vi "Drop Parameters.vi"(6 "Main UI Message Queue":refnum<queue>, 7 "Mouse Position":cluster{"X":i32, "Y":i32}, 8 "error in (no error)":errorcluster, 9 "Parent Window Title":string, 10 "Module Type":T1=enum."Feed", 11 "State in":T2 {"Main Config"."PR Module Configs"."Settings"."PID 2 Parameters"."output range"."output low" format="%.2f"; "Main Config"."PR Module Configs"."Settings"."PID 2 Parameters"."output range"."output high" min=0.0 max=100.0 format="%.2f"; "Main Config"."PR Module Configs"."Settings"."PID 2 Parameters"."PID gains"."derivative time (Td, min)" format="%.3f"; "Main Config"."PR Module Configs"."Settings"."PID 2 Parameters"."PID gains"."integral time (Ti, min)" format="%.3f"; "Main Config"."PR Module Configs"."Settings"."PID 2 Parameters"."PID gains"."proportional gain (Kc)" format="%.3f"; "Main Config"."Steps"."Control" items=["Pump %", "Setpoint"]; "Main Config"."TCU Module Configs"."Settings"."Julabo FP-50 Settings"."Pump Power" min=0 max=8 step=1; "Main Config"."TCU Module Configs"."Settings"."Lauda Settings"."Pump Power" min=0 max=8 step=1; "Main Config"."Pump Module Configs"."Settings"."ASIA Pump C"."channel" min=0 max=1 step=1; "Main Config"."Pump Module Configs"."Settings"."Masterflex"."Pump Number" min=1.0 max=20.0 step=1.0; "Main Config"."Pump Module Configs"."Settings"."Ismatech"."Pump Number" min=1.0 max=20.0 step=1.0; "Main Config"."Feed Module Configs"."Settings"."output range"."output low" min=0.0 max=100.0 format="%.2f"; "Main Config"."Feed Module Configs"."Settings"."output range"."output high" format="%.2f"; "Main Config"."Feed Module Configs"."Settings"."PID 2 Parameters"."PID gains"."derivative time (Td, min)" format="%.3f"; "Main Config"."Feed Module Configs"."Settings"."PID 2 Parameters"."PID gains"."integral time (Ti, min)" format="%.3f"; "Main Config"."Feed Module Configs"."Settings"."PID 2 Parameters"."PID gains"."proportional gain (Kc)" format="%.3f"; "Main Config"."Feed Module Configs"."Settings"."ASIA Pump C"."channel" min=0 max=1 step=1; "Main Config"."Feed Module Configs"."Settings"."Ismatech"."Pump Number" min=1.0 max=20.0 step=1.0; "Main Config"."Feed Module Configs"."Settings"."Masterflex"."Pump Number" min=1.0 max=20.0 step=1.0}) -> (0 "error out":errorcluster, 2 "Drop Parameters":T63, 3 "State out":T2 {"Main Config"."PR Module Configs"."Settings"."PID 2 Parameters"."output range"."output low" format="%.2f"; "Main Config"."PR Module Configs"."Settings"."PID 2 Parameters"."output range"."output high" min=0.0 max=100.0 format="%.2f"; "Main Config"."PR Module Configs"."Settings"."PID 2 Parameters"."PID gains"."derivative time (Td, min)" format="%.3f"; "Main Config"."PR Module Configs"."Settings"."PID 2 Parameters"."PID gains"."integral time (Ti, min)" format="%.3f"; "Main Config"."PR Module Configs"."Settings"."PID 2 Parameters"."PID gains"."proportional gain (Kc)" format="%.3f"; "Main Config"."Steps"."Control" items=["Pump %", "Setpoint"]; "Main Config"."TCU Module Configs"."Settings"."Julabo FP-50 Settings"."Pump Power" min=0 max=8 step=1; "Main Config"."TCU Module Configs"."Settings"."Lauda Settings"."Pump Power" min=0 max=8 step=1; "Main Config"."Pump Module Configs"."Settings"."ASIA Pump C"."channel" min=0 max=1 step=1; "Main Config"."Pump Module Configs"."Settings"."Masterflex"."Pump Number" min=1.0 max=20.0 step=1.0; "Main Config"."Pump Module Configs"."Settings"."Ismatech"."Pump Number" min=1.0 max=20.0 step=1.0; "Main Config"."Feed Module Configs"."Settings"."output range"."output low" min=0.0 max=100.0 format="%.2f"; "Main Config"."Feed Module Configs"."Settings"."output range"."output high" format="%.2f"; "Main Config"."Feed Module Configs"."Settings"."PID 2 Parameters"."PID gains"."derivative time (Td, min)" format="%.3f"; "Main Config"."Feed Module Configs"."Settings"."PID 2 Parameters"."PID gains"."integral time (Ti, min)" format="%.3f"; "Main Config"."Feed Module Configs"."Settings"."PID 2 Parameters"."PID gains"."proportional gain (Kc)" format="%.3f"; "Main Config"."Feed Module Configs"."Settings"."ASIA Pump C"."channel" min=0 max=1 step=1; "Main Config"."Feed Module Configs"."Settings"."Ismatech"."Pump Number" min=1.0 max=20.0 step=1.0; "Main Config"."Feed Module Configs"."Settings"."Masterflex"."Pump Number" min=1.0 max=20.0 step=1.0})   [LabVIEW 2018, in "Drag and Drop.lvlib"]
uses:
  Drag and Drop.lvlib
  Drop Parameters Cluster.ctl
  support/Message Queue/Message Cluster.ctl
  <vilib>/Utility/miscctls.llb/LVPoint32TypeDef.ctl
  State Cluster.ctl
  Thumbnail Cluster.ctl
  Object Cluster.ctl
  <vilib>/Utility/miscctls.llb/LVRectTypeDef.ctl
  Object Type Enum.ctl
  <vilib>/Utility/miscctls.llb/LVPositionTypeDef.ctl
  Config Module/Controls/Main Config Cluster.ctl
  OPC/OPC Module Config.ctl
  Scale Module Folder/Measure Instrument/State Enum.ctl
  OPC/OPC Settings.ctl
  OPC/Variable Data Cluster.ctl
  <vilib>/OPCUA/controls/NodeId.ctl
  <vilib>/OPCUA/controls/OPC UA StatusCode.ctl
  <vilib>/OPCUA/controls/Subscription ID.ctl
  <vilib>/OPCUA/controls/OPC UA Client Refnum.ctl
  <vilib>/OPCUA/controls/Subscription Data Change.ctl
  <vilib>/OPCUA/controls/Data Type.ctl
  Feed Module/Controls/Feed Module Config Cluster.ctl
  Feed Module/Controls/Feed Module Settings Cluster.ctl
  Ismatec ISM 831C/Controls/Ismatech Settings Cluster.ctl
  Masterflex 7550-30/Controls/Settings Cluster.ctl
  Mettler Toledo/Controls/Settings Cluster.ctl
  Bronkhorst M13 Flow Meter/Settings Cluster.ctl
  Measure Instrument/PID 2 Parameters Cluster.ctl
  Measure Instrument/PID Input Enum.ctl
  Measure Instrument/PID 2 Output Enum.ctl
  Tacmina QI/Tacmina QI DAQ Setting.ctl
  KNF Pump/Settings Cluster plus SIMDOS.ctl
  ASIA Pump/Pump Settings.ctl
  VICI M50 Party Mode/Settings Cluster.ctl
  FLOM Pump/Settings Cluster.ctl
  SSI PR Class/SSI PR Settings Cluster.ctl
  TT Module/Controls/TT Module Config Cluster.ctl
  Acquisition/Hardware Configuration.ctl
  Acquisition/Task Cluster.ctl
  PT Module/Controls/PT Module Config Cluster.ctl
  Scale Module Folder/Feed Module/Controls/Scale Module Config Cluster.ctl
  Scale Module Folder/Feed Module/Controls/Scale Module Settings Cluster.ctl
  Pump Module Folder/Pump Module Config Cluster.ctl
  Pump Module Folder/Pump Module Settings Cluster.ctl
  LabJack Module/Controls/U3 Module Config Cluster.ctl
  Decoration Module/Decoration Module Config Cluster.ctl
  Flow Module Folder/Feed Module/Controls/Flow Module Config Cluster.ctl
  Flow Module Folder/Feed Module/Controls/Flow Module Settings Cluster.ctl
  TCU Module/TCU Module Folder/TCU Module Config Cluster.ctl
  TCU Module/TCU Module Folder/TCU Module Settings Cluster.ctl
  TCU Module/TCU Module Folder/Measure Instrument/Output Devices.ctl
  Huber TCU/Huber Settings.ctl
  Lauda Integral XT-150 TCU/Lauda Settings.ctl
  Julabo Type 1 TCU/Julabo Type 1 TCU Folder/Julabo FP-50 Settings.ctl
  Huber Unistat 410 TCU/Huber Unistat 410 Settings.ctl
  D-O Module Folder/Not Sure Where this is Used.ctl
  Sequencing/Squence Control.ctl
  D-O Module Folder/D-O Module Config Cluster.ctl
  D-O Module Folder/Valve Clusters.ctl
  D-O Module Folder/D-O Module Settings Cluster.ctl
  D-O Module Folder/D-O Device Settings Cluster.ctl
  VICI Electronic Actuator/VICI Electronic Actuator Settings.ctl
  Pressure Regulator Control Module/Pressure Regulator/Controls/4-20mA Module Config Cluster.ctl
  Pressure Regulator Control Module/Pressure Regulator/Controls/4-20mA Module Settings Cluster.ctl
  Pressure Transmitter/Pressure Transmitter Device Settings.ctl
  Pressure Reg Module/Pressure Regulator Device Settings.ctl
  Module Type Enum.ctl
  Module Instance Number Operation Enum.ctl
  Flow Module Folder/Flow Module (Main).vi
  D-O Module Folder/D-O Module (Main).vi
  TCU Module/TCU Module Folder/TCU Module (Main).vi
  LabJack Module/U3 (Main).vit
  Feed Module/Feed Module.lvlib
  TT Module/TT Module.lvlib
  support/Message Queue/Message Queue.lvlib
  Bronkhorst M13 Flow Meter/Bronkhorst M13 Flow Meter.lvlib
  Mettler Toledo/Mettler Toledo.lvlib
  Masterflex 7550-30/Masterflex 7550-30.lvlib
  Ismatec ISM 831C/Ismatec ISM 831C.lvlib
  PT Module/PT Module.lvlib
  Shared Variables/Dynamic Shared Variables.lvlib
  Scale Module Folder/Scale Module.lvlib
  Pump Module Folder/Pump Module.lvlib
  LabJack Module/U3 Module.lvlib
  Flow Module Folder/Flow Module.lvlib
  Tacmina QI/Tacmina QI.lvlib
  KNF Pump/KNF SIMDOS.lvlib
  TCU Module/TCU Module Folder/TCU Module.lvlib
  Huber TCU/Huber Ministat 230 TCU.lvlib
  Lauda Integral XT-150 TCU/Lauda TCU.lvlib
  Julabo Type 1 TCU/Julabo Type 1 TCU Folder/Julabo Type FP-50 TCU.lvlib
  ASIA Pump.lvlib
  VICI M50 Party Mode/VICI M6 M50 Party Mode.lvlib
  D-O Module Folder/D-O Module.lvlib
  Pressure Regulator Control Module/Pressure Regulator/4-20mA Module.lvlib
  Pressure Transmitter/Pressure Transmitter Library.lvlib
  Pressure Reg Module/Pressure Regulator Library.lvlib
  FLOM Pump/FLOM Pump.lvlib
  SSI PR Class/SSI PR Pump.lvlib
  Huber Unistat 410 TCU/Huber Unistat 410 TCU.lvlib
  OPC/OPC UA.lvlib
  Scale Module Folder/Measure Instrument/Scale Module Engine.lvlib
  D-O Module Folder/DIO Valve/VICI Electronic Actuator.lvlib
  D-O Module Folder/D-O Module (Main) 2nd.vi
  Config Module/Config Module.lvlib
  DAQ/DAQ.lvlib
  Sequencing/Sequencing Library.lvlib
panel:
  # "Instrument Settings"
  # "Instrument Settings"
  # "Output Instruments"
  # "Flow Meter Settings"
  # "Output Instruments"
  # "Scale Settings"
  # "Output Instruments"
  # "Input Instruments"
  # "Instrument Settings"
  # "Instrument Settings"
  # "Output Instruments"
  # "Flow Meter Settings"
  # "Output Instruments"
  # "Scale Settings"
  # "Output Instruments"
  # "Input Instruments"
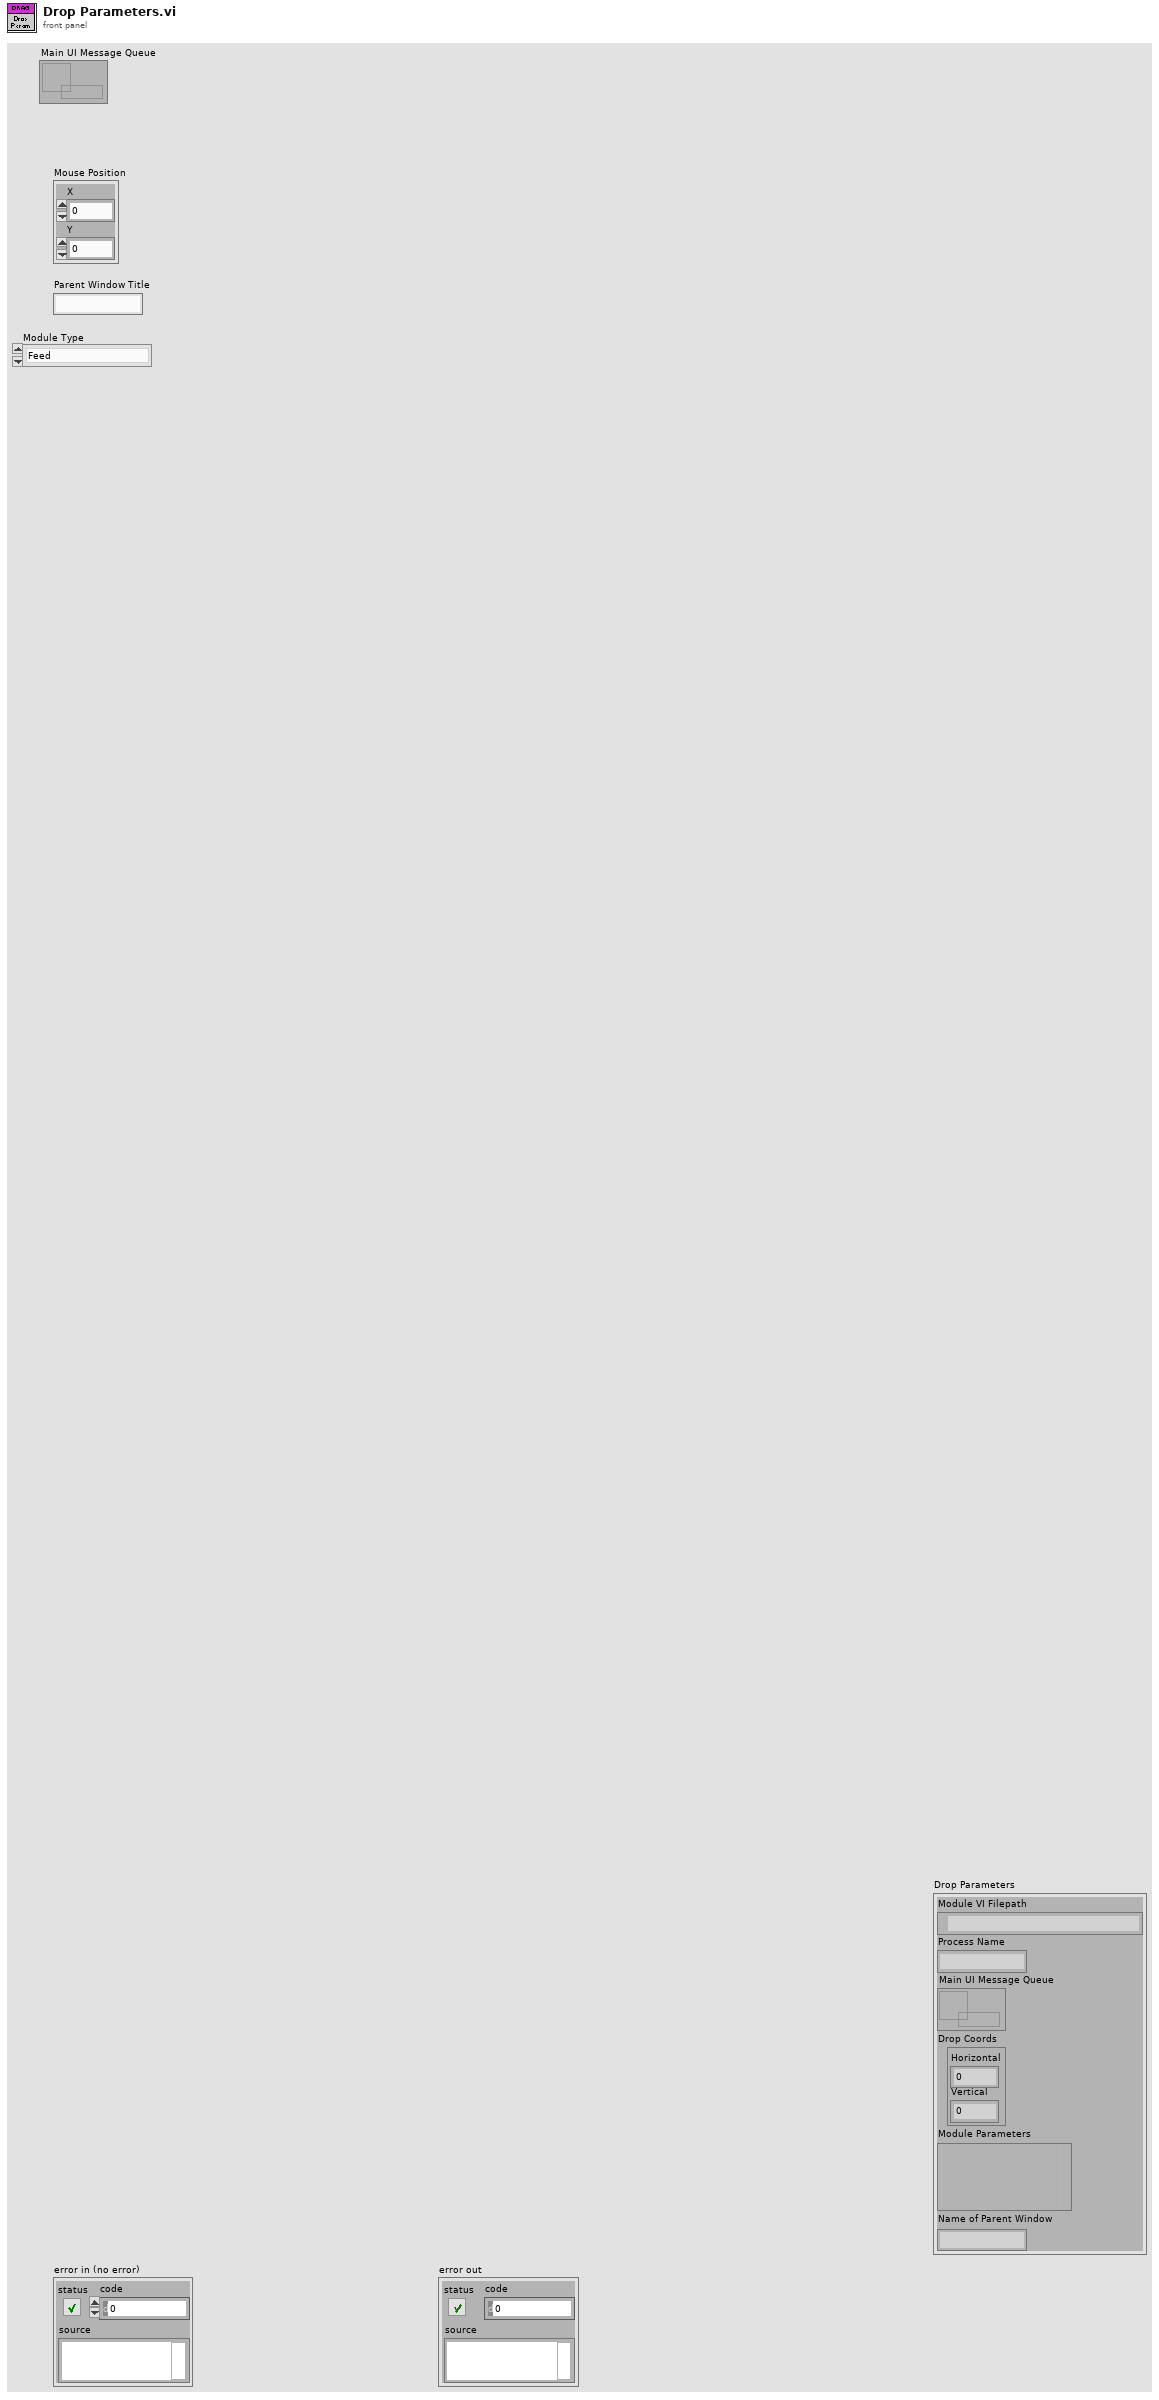
[diagram p1: front panel]
types:
  T1 = typedef "Drag and Drop.lvlib/Module Type Enum.ctl" = enum16{"<unknown module>", "Feed", "TT", "PT", "Scale", "Flow", "Pump", "U3", "TCU", "DO", "PR", "OPC"}
  T2 = typedef "Drag and Drop.lvlib/State Cluster.ctl" = cluster{"VI refs":refnum<vi>[], "Queues":refnum<queue>[], "[Thumbnails]":T3[], "Drag Object Idx":i32, "[Objects]":T4[], "Active Object":i32, "Drop Offset":T7, "Process Name":string, "Main Config":T8, "Campaign Filepath":path, "Config Changed?":bool}
  T3 = typedef "Thumbnail Cluster.ctl" = cluster{"Path":path, "Rectangle":cluster{"left":i16, "top":i16, "right":i16, "bottom":i16}}
  T4 = typedef "Object Cluster.ctl" = cluster{"BMP Path":path, "Anchor Position":cluster{"X":i32, "Y":i32}, "Hot Spot":T5, "Type":T6, "Parameters":variant}
  T5 = typedef "LVRectTypeDef.ctl" = cluster{"Left":i16, "Top":i16, "Right":i16, "Bottom":i16}
  T6 = typedef "Object Type Enum.ctl" = enum16{"Icon", "Line", "Text", "Feed Module"}
  T7 = typedef "LVPositionTypeDef.ctl" = cluster{"Left":i32, "Top":i32}
  T8 = typedef "Config Module.lvlib/Main Config Cluster.ctl" = cluster{"OPC Module Configs":T9[], "Feed Module Configs":T18[], "Log File Path":path, "TT Module Configs":T33[], "DAQ Config":T34, "PT Module Configs":T36[], "Scale Module Configs":T37[], "Pump Module Configs":T39[], "U3 Module Configs":T41[], "Decoration Module Configs":T42[], "Flow Module Configs":T43[], "TCU Module Configs":T45[], "Steps":T52, "Abort":bool, "DO Module Configs":T54[], "PR Module Configs":T59[], "Cycle Period":dbl}
  T9 = typedef "OPC UA.lvlib/OPC Module Config.ctl" = cluster{"State":T10, "GUID":string, "Drop Coords":T11, "Configuration":T12, "First Iteration":bool, "Data":cluster{"Object Name":string, "Variable Array":T13[]}[], "Process Name":string, "Load Count":i32, "Log Started":bool, "subscription ID out":T16, "OPC UA client refnum out":T17, "Event Registration Refnum":refnum<event-registration>, "Start Time":timestamp, "Current Time":timestamp}
  T10 = typedef "Scale Module.lvlib/Scale Module Engine.lvlib/State Enum.ctl" = enum16{"Measuring", "Idle"}
  T11 = typedef "LVPoint32TypeDef.ctl" = cluster{"Horizontal":i32, "Vertical":i32}
  T12 = typedef "OPC UA.lvlib/OPC Settings.ctl" = cluster{"Cycle Period":dbl, "server endpoint URL":string, "security policy":cluster{"message mode":enum16{"None", "Sign", "Sign and Encrypt"}, "security":enum16{"Basic256", "Basic128Rsa15"}}, "Trust Any Server":bool}
  T13 = typedef "OPC UA.lvlib/Variable Data Cluster.ctl" = cluster{"node ID":T14, "browse name":string, "status":T15, "timestamp":timestamp, "value ":variant}
  T14 = typedef "NodeId.ctl" = string
  T15 = typedef "OPC UA StatusCode.ctl" = u32
  T16 = typedef "Subscription ID.ctl" = u32
  T17 = typedef "OPC UA Client Refnum.ctl" = refnum<k21>
  T18 = typedef "Feed Module.lvlib/Feed Module Config Cluster.ctl" = cluster{"GUID":string, "Drop Coords":T11, "Process Name":string, "Queue Name":string, "Settings":T19, "Settings Load Count":i32, "OP Load Count":i32}
  T19 = typedef "Feed Module.lvlib/Feed Module Settings Cluster.ctl" = cluster{"Cycle Period":dbl, "Ismatech":T20, "Masterflex":T21, "Mettler":T22, "Bronkhorst M13 Flow Meter":T23, "PID 2 Parameters":T24, "Manual Entry":dbl, "Auto?":bool, "output range":cluster{"output high":dbl, "output low":dbl}, "Bronkhorst M14":T22, "Tacmina Settings":T27, "KNF SIMDOS Settings":T28, "ASIA Pump C":T29, "VICI Settings":T30, "FLOM Settings":T31, "SSI PR Settings":T32}
  T20 = typedef "Ismatec ISM 831C.lvlib/Ismatech Settings Cluster.ctl" = cluster{"VISA resource name":refnum<visa-resource-name>, "Simulated?":bool, "Pump Number":dbl, "Reverse?":bool}
  T21 = typedef "Masterflex 7550-30.lvlib/Settings Cluster.ctl" = cluster{"VISA resource name":refnum<visa-resource-name>, "Simulated?":bool, "Pump Number":dbl, "Reverse?":bool}
  T22 = typedef "Mettler Toledo.lvlib/Settings Cluster.ctl" = cluster{"VISA resource name":refnum<visa-resource-name>, "Simulated?":bool}
  T23 = typedef "Bronkhorst M13 Flow Meter.lvlib/Settings Cluster.ctl" = cluster{"VISA resource name":refnum<visa-resource-name>, "Simulated?":bool}
  T24 = typedef "PID 2 Parameters Cluster.ctl" = cluster{"Input Device":T25, "Output Device":T26, "Setpoint":dbl, "PID gains":cluster{"proportional gain (Kc)":dbl, "integral time (Ti, min)":dbl, "derivative time (Td, min)":dbl}}
  T25 = typedef "PID Input Enum.ctl" = enum16{"Default", "Bronkhorst M13", "Bronkhorst M14", "Scale Rate of Change"}
  T26 = typedef "PID 2 Output Enum.ctl" = enum16{"Default", "Ismatec ISM 831C", "Masterflex 7550-30", "VICI", "Tacmina QI", "KNF SIMDOS", "ASIA Type C", "FLOM UI-22-11", "SSI PR"}
  T27 = typedef "Tacmina QI.lvlib/Tacmina QI DAQ Setting.ctl" = cluster{"Analog DAQ Task":refnum<k21>, "Digital DAQ Task":refnum<k21>}
  T28 = typedef "KNF SIMDOS.lvlib/Settings Cluster plus SIMDOS.ctl" = cluster{"VISA resource name":refnum<visa-resource-name>, "Simulated?":bool}
  T29 = typedef "ASIA Pump.lvlib/Pump Settings.ctl" = cluster{"ASIA Pump #":i32, "channel":i32, "Simulated":bool}
  T30 = typedef "VICI M6 M50 Party Mode.lvlib/Settings Cluster.ctl" = cluster{"VISA resource name":refnum<visa-resource-name>, "Simulated?":bool, "Pump Letter":string, "Reverse?":bool}
  T31 = typedef "FLOM Pump.lvlib/Settings Cluster.ctl" = cluster{"VISA resource name":refnum<visa-resource-name>, "Simulated?":bool, "Pump Number":dbl}
  T32 = typedef "SSI PR Pump.lvlib/SSI PR Settings Cluster.ctl" = cluster{"VISA resource name":refnum<visa-resource-name>, "Simulated?":bool}
  T33 = typedef "TT Module.lvlib/TT Module Config Cluster.ctl" = cluster{"GUID":string, "Drop Coords":T11, "Input Channel Tag Name ":string, "Process Name":string, "Queue Name":string, "Input Channel Numeric Alarm Settings":cluster{"enable? (F)":bool, "name":string, "alarm type":enum16{"HI_HI", "HI", "LO", "LO_LO"}, "level/change":dbl, "deadband/time":dbl, "priority":u32, "ack type":enum16{"Auto", "User", "None", "Each Occurrence"}, "area":string, "description":string, "log? (T)":bool}[]}
  T34 = typedef "DAQ.lvlib/Hardware Configuration.ctl" = cluster{"Tasks":T35[]}
  T35 = typedef "Task Cluster.ctl" = cluster{"DAQmx Task":refnum<k21>, "Read-Write Radio":enum32{"Read", "Write"}}
  T36 = typedef "PT Module.lvlib/PT Module Config Cluster.ctl" = cluster{"GUID":string, "Drop Coords":T11, "Input Channel Tag Name ":string, "Process Name":string, "Queue Name":string, "Input Channel Numeric Alarm Settings":cluster{"enable? (F)":bool, "name":string, "alarm type":enum16{"HI_HI", "HI", "LO", "LO_LO"}, "level/change":dbl, "deadband/time":dbl, "priority":u32, "ack type":enum16{"Auto", "User", "None", "Each Occurrence"}, "area":string, "description":string, "log? (T)":bool}[]}
  T37 = typedef "Scale Module.lvlib/Scale Module Config Cluster.ctl" = cluster{"GUID":string, "Drop Coords":T11, "Process Name":string, "Queue Name":string, "Settings":T38, "Load Count":i32}
  T38 = typedef "Scale Module.lvlib/Scale Module Settings Cluster.ctl" = cluster{"Cycle Period":dbl, "Mettler":T22, "Scale Type":string}
  T39 = typedef "Pump Module.lvlib/Pump Module Config Cluster.ctl" = cluster{"GUID":string, "Drop Coords":T11, "Process Name":string, "Queue Name":string, "Settings":T40, "Load Count":i32}
  T40 = typedef "Pump Module.lvlib/Pump Module Settings Cluster.ctl" = cluster{"Cycle Period":dbl, "Ismatech":T20, "Masterflex":T21, "Manual Entry":dbl, "VICI Settings":T30, "Output Device":T26, "Tacmina Settings":T27, "KNF SIMDOS Settings":T28, "ASIA Pump C":T29, "FLOM Settings":T31, "Pump Calibration File":path, "Calibration":dbl, "Pump Cal Enum":u16, "SSI PR Settings":T32}
  T41 = typedef "U3 Module.lvlib/U3 Module Config Cluster.ctl" = cluster{"GUID":string, "Drop Coords":T11, "AI Channel Number":enum16{"Default", "AI0", "AI1", "AI2", "AI3", "AI4", "AI5", "AI6", "AI7"}, "Process Name":string, "Queue Name":string, "Input Channel Numeric Alarm Settings":cluster{"enable? (F)":bool, "name":string, "alarm type":enum16{"HI_HI", "HI", "LO", "LO_LO"}, "level/change":dbl, "deadband/time":dbl, "priority":u32, "ack type":enum16{"Auto", "User", "None", "Each Occurrence"}, "area":string, "description":string, "log? (T)":bool}[]}
  T42 = typedef "Decoration Module Config Cluster.ctl" = cluster{"GUID":string, "Drop Coords":T11, "Decoration Filepath":path}
  T43 = typedef "Flow Module.lvlib/Flow Module Config Cluster.ctl" = cluster{"GUID":string, "Drop Coords":T11, "Process Name":string, "Queue Name":string, "Settings":T44, "Load Count":i32}
  T44 = typedef "Flow Module.lvlib/Flow Module Settings Cluster.ctl" = cluster{"Cycle Period":dbl, "Bronkhorst M13":T22, "Flow Meter Type":string, "Bronkhorst M14":T22}
  T45 = typedef "TCU Module.lvlib/TCU Module Config Cluster.ctl" = cluster{"GUID":string, "Drop Coords":T11, "Process Name":string, "Queue Name":string, "Settings":T46, "Load Count":i32, "Power Level Changed":bool}
  T46 = typedef "TCU Module.lvlib/TCU Module Settings Cluster.ctl" = cluster{"Cycle Period":dbl, "Setpoint Entry":dbl, "Output Device":T47, "Huber Ministat 230 Settings":T48, "Lauda Settings":T49, "Julabo FP-50 Settings":T50, "Internal Control?":bool, "Huber Unistat 410 Settings":T51}
  T47 = typedef "Output Devices.ctl" = enum16{"Default", "Huber Ministat 230", "Huber Unistat 410", "Lauda XT-150", "Julabo FP-50"}
  T48 = typedef "Huber Ministat 230 TCU.lvlib/Huber Settings.ctl" = cluster{"VISA resource name":refnum<visa-resource-name>, "Simulated?":bool}
  T49 = typedef "Lauda TCU.lvlib/Lauda Settings.ctl" = cluster{"VISA resource name":refnum<visa-resource-name>, "Simulated?":bool, "Pump Power":i32}
  T50 = typedef "Julabo Type FP-50 TCU.lvlib/Julabo FP-50 Settings.ctl" = cluster{"VISA resource name":refnum<visa-resource-name>, "Simulated?":bool, "Pump Power":i32}
  T51 = typedef "Huber Unistat 410 TCU.lvlib/Huber Unistat 410 Settings.ctl" = cluster{"VISA resource name":refnum<visa-resource-name>, "Simulated?":bool}
  T52 = typedef "Not Sure Where this is Used.ctl" = T53[]
  T53 = typedef "Sequencing Library.lvlib/Squence Control.ctl" = cluster{"Module":string, "Control":u16, "Value":dbl, "Wait (sec)":dbl}
  T54 = typedef "D-O Module.lvlib/D-O Module Config Cluster.ctl" = cluster{"GUID":string, "Drop Coords":T11, "Process Name":string, "Queue Name":string, "Settings":T55, "Load Count":i32}
  T55 = typedef "D-O Module.lvlib/Valve Clusters.ctl" = cluster{"Valve Settings":T56, "Valve Type":enum16{"Default", "Digital Output Valve", "VICI Electronic Actuator"}, "Time On (Sec)":dbl, "Time Off (Sec)":dbl, "Run?":bool}
  T56 = typedef "D-O Module.lvlib/D-O Module Settings Cluster.ctl" = cluster{"D-O Settings":T57, "VICI Electronic Actuator":T58}
  T57 = typedef "D-O Module.lvlib/D-O Device Settings Cluster.ctl" = cluster{"DAQmx Task Name":refnum<k21>, "Output Channel":u16, "Output Channel Names":string[]}
  T58 = typedef "VICI Electronic Actuator.lvlib/VICI Electronic Actuator Settings.ctl" = cluster{"VISA resource name":refnum<visa-resource-name>, "Mode":enum16{"Two Positions With Stops", "Two Positions Without Stops", "Mutiposition"}, "Simulated":bool}
  T59 = typedef "4-20mA Module.lvlib/4-20mA Module Config Cluster.ctl" = cluster{"GUID":string, "Drop Coords":T11, "Process Name":string, "Queue Name":string, "Settings":T60, "Settings Load Count":i32}
  T60 = typedef "4-20mA Module.lvlib/4-20mA Module Settings Cluster.ctl" = cluster{"Cycle Period":dbl, "PID 2 Parameters":cluster{"Input Device":enum16{"Default", "4-20mA"}, "Output Device":enum16{"Default", "Equilibar Pressure Reg", "Flow Regulator"}, "Setpoint":dbl, "PID gains":cluster{"proportional gain (Kc)":dbl, "integral time (Ti, min)":dbl, "derivative time (Td, min)":dbl}, "output range":cluster{"output low":dbl, "output high":dbl}}, "Manual Entry":dbl, "Auto?":bool, "4-20mA Input Settings":T61, "4-20mA Out Settings":T62, "Input Channel Tag Name ":string}
  T61 = typedef "Pressure Transmitter Library.lvlib/Pressure Transmitter Device Settings.ctl" = cluster{"Input Channel ":u16}
  T62 = typedef "Pressure Regulator Library.lvlib/Pressure Regulator Device Settings.ctl" = cluster{"Output DAQ Task":refnum<k21>}
  T63 = typedef "Drop Parameters Cluster.ctl" = cluster{"Module VI Filepath":path, "Process Name":string, "Main UI Message Queue":refnum<queue>, "Drop Coords":T11, "Module Parameters":variant, "Name of Parent Window":string}
  T64 = typedef "Module Instance Number Operation Enum.ctl" = enum16{"Init", "Next Instance Number"}
  T65 = cluster{"enable? (F)":bool, "name":string, "alarm type":enum16{"HI_HI", "HI", "LO", "LO_LO"}, "level/change":dbl, "deadband/time":dbl, "priority":u32, "ack type":enum16{"Auto", "User", "None", "Each Occurrence"}, "area":string, "description":string, "log? (T)":bool}[]
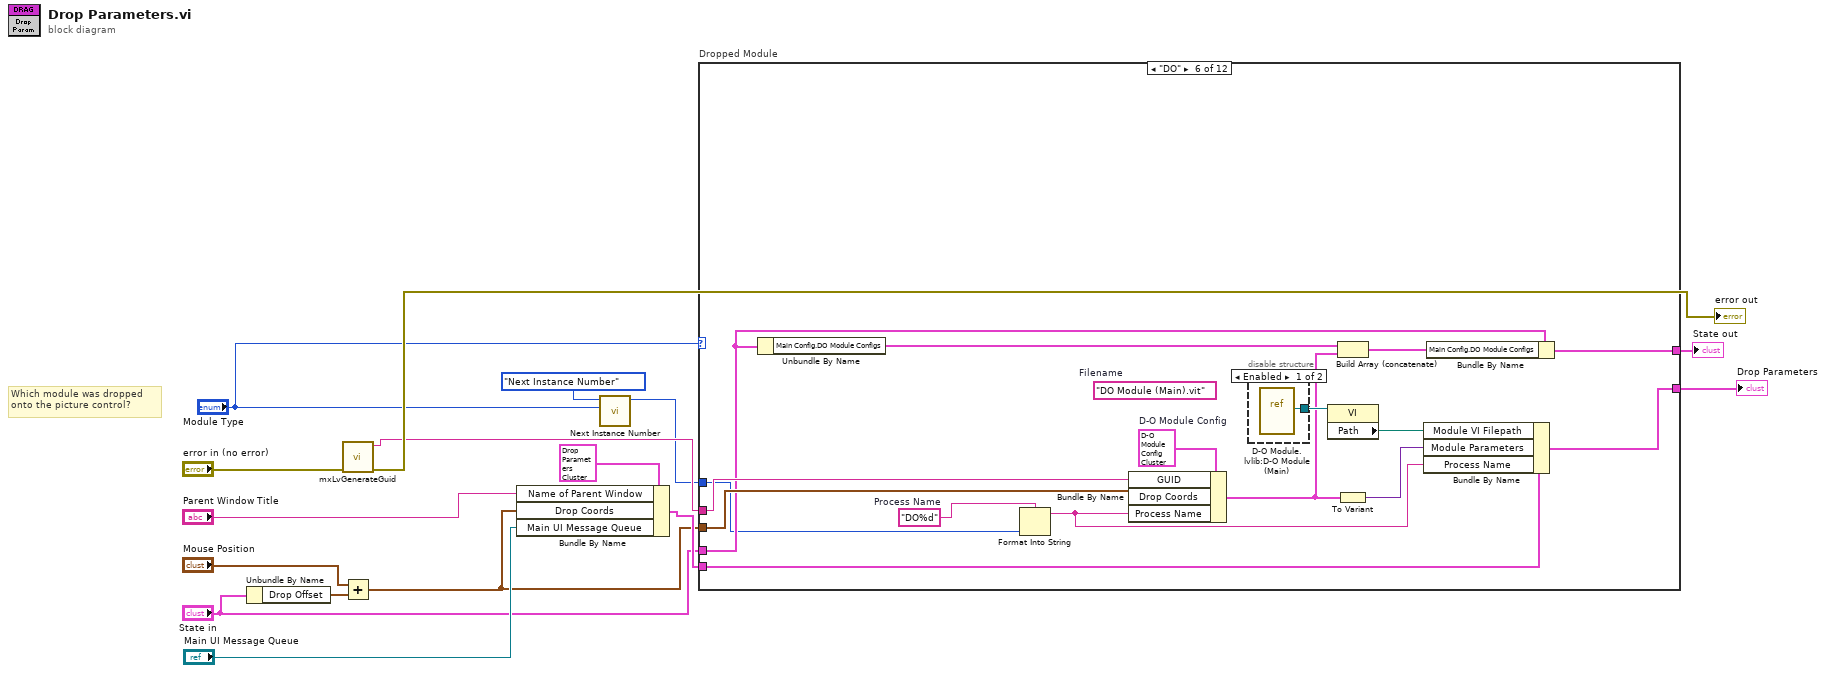
[diagram p0: block diagram]
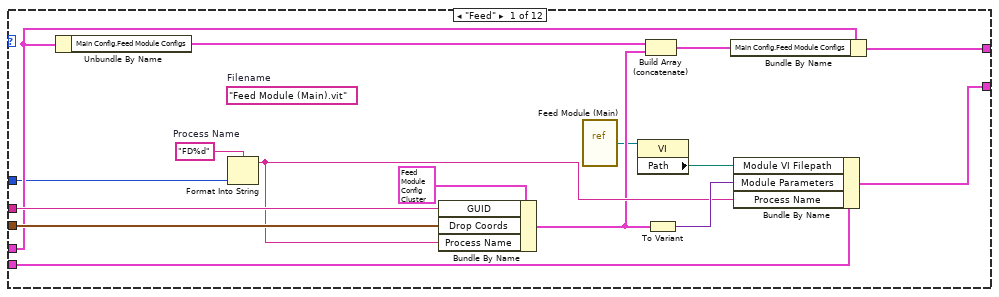
[diagram p2: hidden frame]
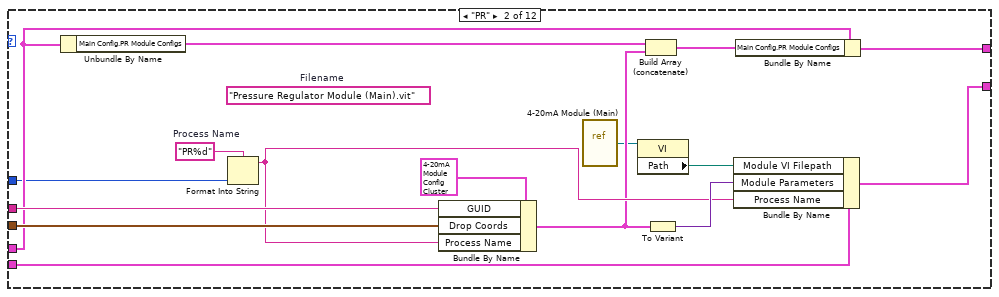
[diagram p3: hidden frame]
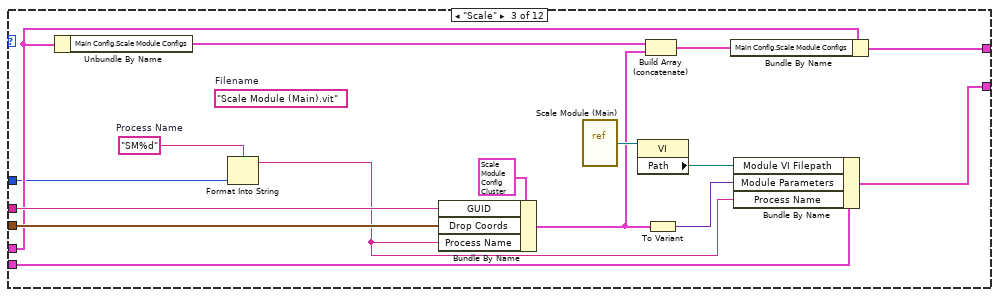
[diagram p4: hidden frame]
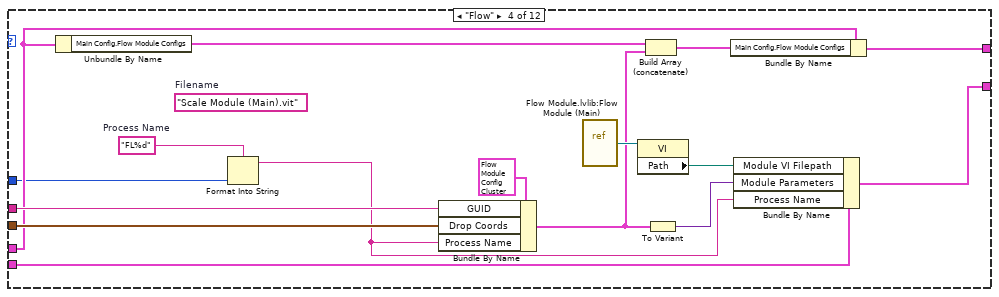
[diagram p5: hidden frame]
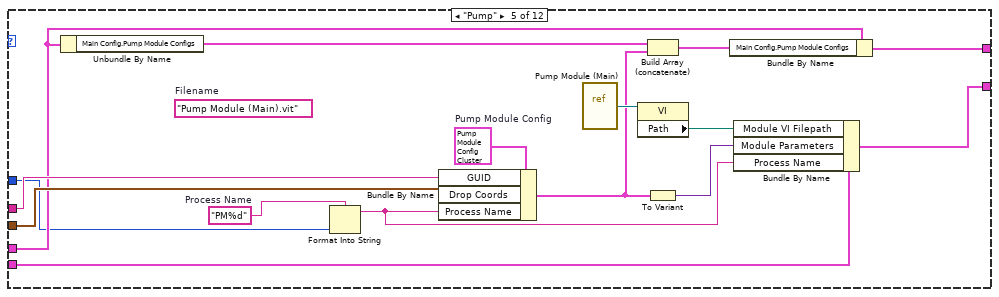
[diagram p6: hidden frame]
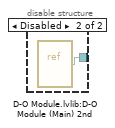
[diagram p7: hidden frame]
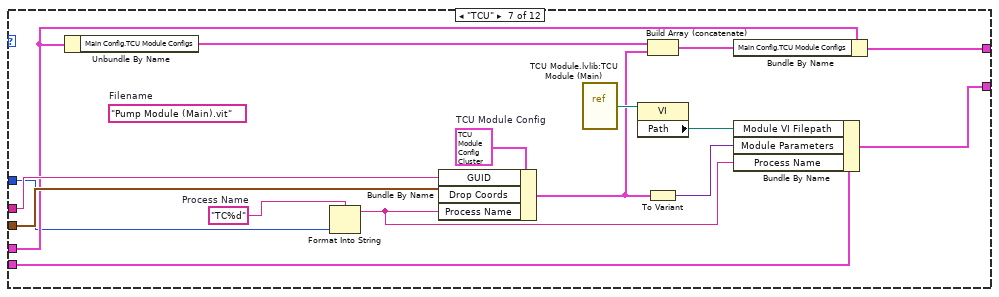
[diagram p8: hidden frame]
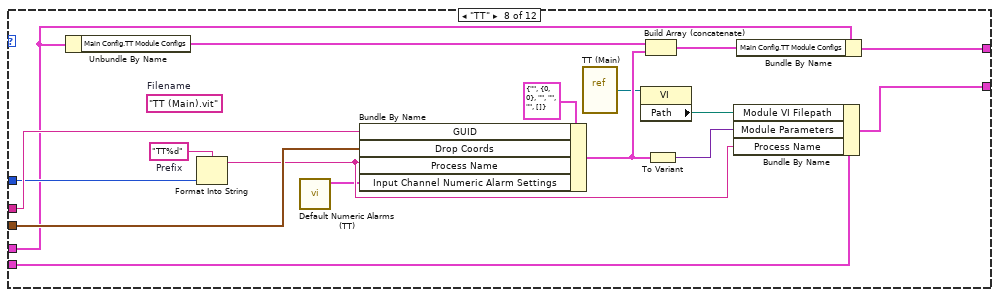
[diagram p9: hidden frame]
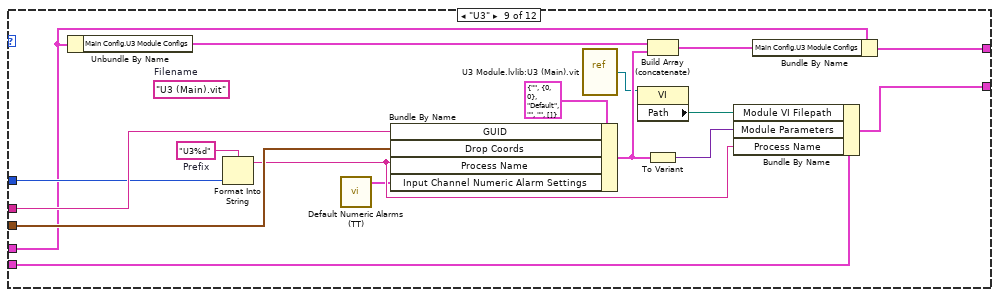
[diagram p10: hidden frame]
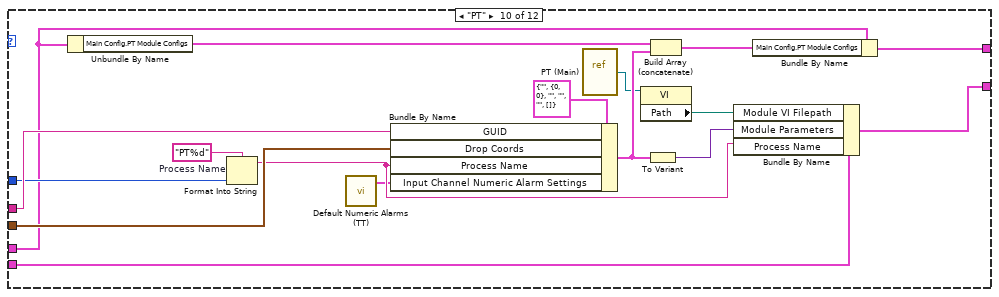
[diagram p11: hidden frame]
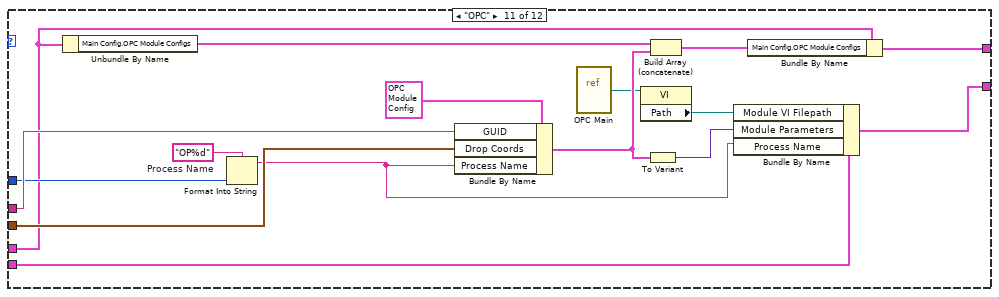
[diagram p12: hidden frame]
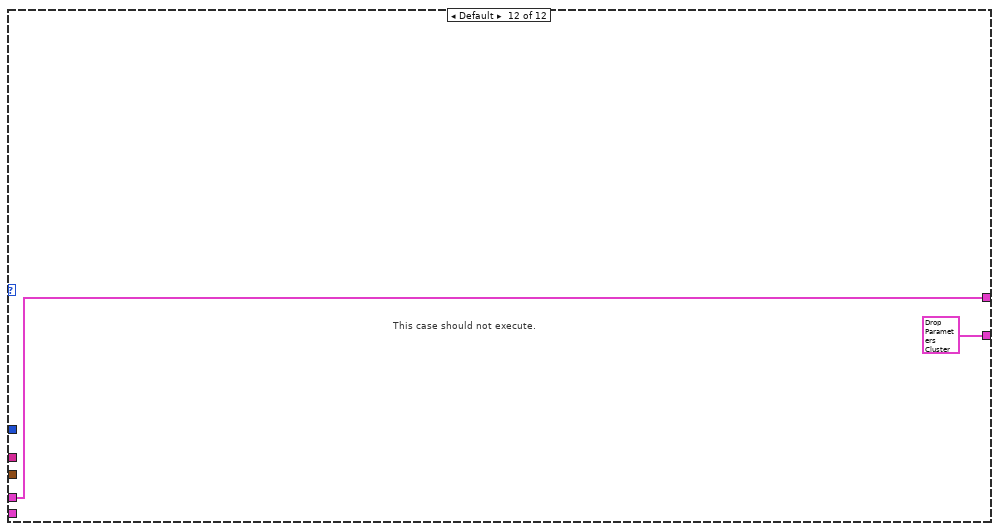
[diagram p13: hidden frame]
diagram:
  # "Which module was dropped\nonto the picture control?"
  n1 = Unbundle By Name("State in") -> ("Drop Offset"=w12:T7)
  n2 = call <resource>:"mxLvGenerateGuid.vi"("Error In"="error in (no error)") -> ("Error Out"=→"error out":errorcluster, "Value"=w13:string)  [unwired: 9 in]
  n3 = Add(x="Mouse Position", y=w12) -> (x+y=w6:T7)
  n4 = Bundle By Name(cluster=T63 {"Module VI Filepath"=path "", "Process Name"="", "Main UI Message Queue"=refnum, "Drop Coords"={"Horizontal"=0, "Vertical"=0}, "Module Parameters"=variant, "Name of Parent Window"=""} ("Drop Parameters"), "Name of Parent Window"="Parent Window Title", "Drop Coords"=w6, "Main UI Message Queue"="Main UI Message Queue") -> (w8:T63)
  n5 = call "Next Instance Number.vi"("Module Type"="Module Type", "Operation"=Module_Instance_Number_Operation_Enum."Next Instance Number") -> ("Instance Number"=w3:i32)  [unwired: 8 in, 1 out]
  n6 = case "Dropped Module" shown="\"DO\"" "Module Type" {
    tunnel: "State in" -> [w18 w34 w51 w67 w84 w100 w118 w132 w149 w166 w185 w199]
    tunnel: [w24 w40 w56 w72 w89 w105 w123 w136 w153 w170 w188 w199] -> w2
    tunnel: [w30 w46 w62 w78 w95 w111 w129 w146 w163 w180 w182 T63 {"Module VI Filepath"=path "", "Process Name"="", "Main UI Message Queue"=refnum, "Drop Coords"={"Horizontal"=0, "Vertical"=0}, "Module Parameters"=variant, "Name of Parent Window"=""} ("Drop Parameters")] -> w16
    tunnel: w13 -> [w29 w45 w61 w77 w94 w110 w128 w145 w162 w179 w196 _]
    tunnel: w8 -> [w28 w44 w60 w76 w93 w109 w127 w144 w161 w178 w195 _]
    tunnel: w6 -> [w26 w42 w58 w74 w91 w107 w125 w142 w159 w176 w193 _]
    tunnel: w3 -> [w17 w33 w50 w66 w83 w99 w117 w133 w150 w167 w186 _]
    frame "Feed" {
      w31 = "FD%d"  # Process Name
      (unwired) "Feed Module (Main).vit"  # Filename
      n7 = Unbundle By Name(w18) -> ("Main Config.Feed Module Configs"=w23:T18[])
      n8 = Format Into String(format string=w31, w17) -> (resulting string=w25:string)  [unwired: 2 in, 1 out]
      n9 = Bundle By Name(cluster=T18 {"GUID"="", "Drop Coords"={"Horizontal"=0, "Vertical"=0}, "Process Name"="", "Queue Name"="", "Settings"={"Cycle Period"=500.0, "Ismatech"={"VISA resource name"="", "Simulated?"=TRUE, "Pump Number"=1.0, "Reverse?"=FALSE}, "Masterflex"={"VISA resource name"="", "Simulated?"=TRUE, "Pump Number"=1.0, "Reverse?"=FALSE}, "Mettler"={"VISA resource name"="", "Simulated?"=FALSE}, "Bronkhorst M13 Flow Meter"={"VISA resource name"="", "Simulated?"=TRUE}, "PID 2 Parameters"={"Input Device"=enum."Default", "Output Device"=enum."Default", "Setpoint"=0.0, "PID gains"={"proportional gain (Kc)"=1.0, "integral time (Ti, min)"=0.01, "derivative time (Td, min)"=0.0}}, "Manual Entry"=0.0, "Auto?"=TRUE, "output range"={"output high"=100.0, "output low"=0.0}, "Bronkhorst M14"={"VISA resource name"="", "Simulated?"=FALSE}, "Tacmina Settings"={"Analog DAQ Task"="", "Digital DAQ Task"=""}, "KNF SIMDOS Settings"={"VISA resource name"="", "Simulated?"=TRUE}, "ASIA Pump C"={"ASIA Pump #"=0, "channel"=0, "Simulated"=FALSE}, "VICI Settings"={"VISA resource name"="", "Simulated?"=TRUE, "Pump Letter"="", "Reverse?"=FALSE}, "FLOM Settings"={"VISA resource name"="", "Simulated?"=TRUE, "Pump Number"=0.0}, "SSI PR Settings"={"VISA resource name"="", "Simulated?"=FALSE}}, "Settings Load Count"=0, "OP Load Count"=0} ("Feed Module Config"), "GUID"=w29, "Drop Coords"=w26, "Process Name"=w25) -> (w21:T18)
      n10 = vi-ref "Feed Module (Main).vi"() -> (w20:refnum<vi>)
      n11 = property class="VI"(reference=w20) -> ("Path"=w19:path)  [unwired: 1 in, 2 out]
      n12 = Build Array (concatenate)(w23, w21) -> (w22:T18[])
      n13 = To Variant(anything=w21) -> (Variant=w27:variant)
      n14 = Bundle By Name(cluster=w18, "Main Config.Feed Module Configs"=w22) -> (w24:T2)
      n15 = Bundle By Name(cluster=w28, "Module VI Filepath"=w19, "Module Parameters"=w27, "Process Name"=w25) -> (w30:T63)
    }
    frame "PR" {
      w47 = "PR%d"  # Process Name
      (unwired) "Pressure Regulator Module (Main).vit"  # Filename
      n16 = Unbundle By Name(w34) -> ("Main Config.PR Module Configs"=w39:T59[])
      n17 = Format Into String(format string=w47, w33) -> (resulting string=w41:string)  [unwired: 2 in, 1 out]
      n18 = Bundle By Name(cluster=T59 {"GUID"="", "Drop Coords"={"Horizontal"=0, "Vertical"=0}, "Process Name"="", "Queue Name"="", "Settings"={"Cycle Period"=500.0, "PID 2 Parameters"={"Input Device"=enum."Default", "Output Device"=enum."Default", "Setpoint"=0.0, "PID gains"={"proportional gain (Kc)"=1.0, "integral time (Ti, min)"=0.01, "derivative time (Td, min)"=0.0}, "output range"={"output low"=0.0, "output high"=100.0}}, "Manual Entry"=0.0, "Auto?"=TRUE, "4-20mA Input Settings"={"Input Channel "=0}, "4-20mA Out Settings"={"Output DAQ Task"=""}, "Input Channel Tag Name "=""}, "Settings Load Count"=0} ("PRM Config"), "GUID"=w45, "Drop Coords"=w42, "Process Name"=w41) -> (w37:T59)
      n19 = vi-ref "4-20mA Module (Main).vi"() -> (w36:refnum<vi>)
      n20 = property class="VI"(reference=w36) -> ("Path"=w35:path)  [unwired: 1 in, 2 out]
      n21 = Build Array (concatenate)(w39, w37) -> (w38:T59[])
      n22 = To Variant(anything=w37) -> (Variant=w43:variant)
      n23 = Bundle By Name(cluster=w44, "Module VI Filepath"=w35, "Module Parameters"=w43, "Process Name"=w41) -> (w46:T63)
      n24 = Bundle By Name(cluster=w34, "Main Config.PR Module Configs"=w38) -> (w40:T2)
    }
    frame "Scale" {
      w63 = "SM%d"  # Process Name
      (unwired) "Scale Module (Main).vit"  # Filename
      n25 = Unbundle By Name(w51) -> ("Main Config.Scale Module Configs"=w55:T37[])
      n26 = Format Into String(format string=w63, w50) -> (resulting string=w57:string)  [unwired: 2 in, 1 out]
      n27 = Bundle By Name(cluster=T37 {"GUID"="", "Drop Coords"={"Horizontal"=0, "Vertical"=0}, "Process Name"="", "Queue Name"="", "Settings"={"Cycle Period"=500.0, "Mettler"={"VISA resource name"="", "Simulated?"=TRUE}, "Scale Type"=""}, "Load Count"=0} ("Scale Module Config"), "GUID"=w61, "Drop Coords"=w58, "Process Name"=w57) -> (w49:T37)
      n28 = vi-ref "Scale Module (Main).vi"() -> (w53:refnum<vi>)
      n29 = property class="VI"(reference=w53) -> ("Path"=w52:path)  [unwired: 1 in, 2 out]
      n30 = Build Array (concatenate)(w55, w49) -> (w54:T37[])
      n31 = To Variant(anything=w49) -> (Variant=w59:variant)
      n32 = Bundle By Name(cluster=w51, "Main Config.Scale Module Configs"=w54) -> (w56:T2)
      n33 = Bundle By Name(cluster=w60, "Module VI Filepath"=w52, "Module Parameters"=w59, "Process Name"=w57) -> (w62:T63)
    }
    frame "Flow" {
      w79 = "FL%d"  # Process Name
      (unwired) "Scale Module (Main).vit"  # Filename
      n34 = Unbundle By Name(w67) -> ("Main Config.Flow Module Configs"=w71:T43[])
      n35 = Format Into String(format string=w79, w66) -> (resulting string=w73:string)  [unwired: 2 in, 1 out]
      n36 = Bundle By Name(cluster=T43 {"GUID"="", "Drop Coords"={"Horizontal"=0, "Vertical"=0}, "Process Name"="", "Queue Name"="", "Settings"={"Cycle Period"=500.0, "Bronkhorst M13"={"VISA resource name"="", "Simulated?"=TRUE}, "Flow Meter Type"="", "Bronkhorst M14"={"VISA resource name"="", "Simulated?"=FALSE}}, "Load Count"=0} ("Scale Module Config"), "GUID"=w77, "Drop Coords"=w74, "Process Name"=w73) -> (w65:T43)
      n37 = vi-ref "Flow Module.lvlib:Flow Module (Main).vi"() -> (w69:refnum<vi>)
      n38 = property class="VI"(reference=w69) -> ("Path"=w68:path)  [unwired: 1 in, 2 out]
      n39 = Build Array (concatenate)(w71, w65) -> (w70:T43[])
      n40 = To Variant(anything=w65) -> (Variant=w75:variant)
      n41 = Bundle By Name(cluster=w67, "Main Config.Flow Module Configs"=w70) -> (w72:T2)
      n42 = Bundle By Name(cluster=w76, "Module VI Filepath"=w68, "Module Parameters"=w75, "Process Name"=w73) -> (w78:T63)
    }
    frame "Pump" {
      w81 = T39 {"GUID"="", "Drop Coords"={"Horizontal"=0, "Vertical"=0}, "Process Name"="", "Queue Name"="", "Settings"={"Cycle Period"=500.0, "Ismatech"={"VISA resource name"="", "Simulated?"=TRUE, "Pump Number"=1.0, "Reverse?"=FALSE}, "Masterflex"={"VISA resource name"="", "Simulated?"=TRUE, "Pump Number"=1.0, "Reverse?"=FALSE}, "Manual Entry"=0.0, "VICI Settings"={"VISA resource name"="", "Simulated?"=TRUE, "Pump Letter"="", "Reverse?"=FALSE}, "Output Device"=enum."Default", "Tacmina Settings"={"Analog DAQ Task"="", "Digital DAQ Task"=""}, "KNF SIMDOS Settings"={"VISA resource name"="", "Simulated?"=TRUE}, "ASIA Pump C"={"ASIA Pump #"=0, "channel"=0, "Simulated"=FALSE}, "FLOM Settings"={"VISA resource name"="", "Simulated?"=TRUE, "Pump Number"=0.0}, "Pump Calibration File"=path "", "Calibration"=0.0, "Pump Cal Enum"=0, "SSI PR Settings"={"VISA resource name"="", "Simulated?"=FALSE}}, "Load Count"=0}  # Pump Module Config
      w96 = "PM%d"  # Process Name
      (unwired) "Pump Module (Main).vit"  # Filename
      n43 = Unbundle By Name(w84) -> ("Main Config.Pump Module Configs"=w88:T39[])
      n44 = Format Into String(format string=w96, w83) -> (resulting string=w90:string)  [unwired: 2 in, 1 out]
      n45 = Bundle By Name(cluster=w81, "GUID"=w94, "Drop Coords"=w91, "Process Name"=w90) -> (w82:T39)
      n46 = vi-ref "Pump Module (Main).vi"() -> (w86:refnum<vi>)
      n47 = property class="VI"(reference=w86) -> ("Path"=w85:path)  [unwired: 1 in, 2 out]
      n48 = Build Array (concatenate)(w88, w82) -> (w87:T39[])
      n49 = To Variant(anything=w82) -> (Variant=w92:variant)
      n50 = Bundle By Name(cluster=w84, "Main Config.Pump Module Configs"=w87) -> (w89:T2)
      n51 = Bundle By Name(cluster=w93, "Module VI Filepath"=w85, "Module Parameters"=w92, "Process Name"=w90) -> (w95:T63)
    }
    frame "DO" {
      w97 = T54 {"GUID"="", "Drop Coords"={"Horizontal"=0, "Vertical"=0}, "Process Name"="", "Queue Name"="", "Settings"={"Valve Settings"={"D-O Settings"={"DAQmx Task Name"="", "Output Channel"=0, "Output Channel Names"=[]}, "VICI Electronic Actuator"={"VISA resource name"="", "Mode"=enum."Two Positions With Stops", "Simulated"=FALSE}}, "Valve Type"=enum."Default", "Time On (Sec)"=0.0, "Time Off (Sec)"=0.0, "Run?"=FALSE}, "Load Count"=0}  # D-O Module Config
      w112 = "DO%d"  # Process Name
      (unwired) "DO Module (Main).vit"  # Filename
      n52 = Unbundle By Name(w100) -> ("Main Config.DO Module Configs"=w104:T54[])
      n53 = Format Into String(format string=w112, w99) -> (resulting string=w106:string)  [unwired: 2 in, 1 out]
      n54 = Bundle By Name(cluster=w97, "GUID"=w110, "Drop Coords"=w107, "Process Name"=w106) -> (w98:T54)
      n55 = disable-structure shown="Enabled" {
        disable-tunnel: [w113 w114] -> w102
        frame Enabled {
          n56 = vi-ref "D-O Module.lvlib:D-O Module (Main).vi"() -> (w113:refnum<vi>)
        }
        frame Disabled {
          n57 = vi-ref "D-O Module.lvlib:D-O Module (Main) 2nd.vi"() -> (w114:refnum<vi>)
        }
      }
      n58 = property class="VI"(reference=w102) -> ("Path"=w101:path)  [unwired: 1 in, 2 out]
      n59 = Build Array (concatenate)(w104, w98) -> (w103:T54[])
      n60 = To Variant(anything=w98) -> (Variant=w108:variant)
      n61 = Bundle By Name(cluster=w109, "Module VI Filepath"=w101, "Module Parameters"=w108, "Process Name"=w106) -> (w111:T63)
      n62 = Bundle By Name(cluster=w100, "Main Config.DO Module Configs"=w103) -> (w105:T2)
    }
    frame "TCU" {
      w115 = T45 {"GUID"="", "Drop Coords"={"Horizontal"=0, "Vertical"=0}, "Process Name"="", "Queue Name"="", "Settings"={"Cycle Period"=500.0, "Setpoint Entry"=0.0, "Output Device"=enum."Default", "Huber Ministat 230 Settings"={"VISA resource name"="", "Simulated?"=FALSE}, "Lauda Settings"={"VISA resource name"="", "Simulated?"=FALSE, "Pump Power"=2}, "Julabo FP-50 Settings"={"VISA resource name"="", "Simulated?"=FALSE, "Pump Power"=2}, "Internal Control?"=FALSE, "Huber Unistat 410 Settings"={"VISA resource name"="", "Simulated?"=FALSE}}, "Load Count"=0, "Power Level Changed"=FALSE}  # TCU Module Config
      w130 = "TC%d"  # Process Name
      (unwired) "Pump Module (Main).vit"  # Filename
      n63 = Unbundle By Name(w118) -> ("Main Config.TCU Module Configs"=w122:T45[])
      n64 = Format Into String(format string=w130, w117) -> (resulting string=w124:string)  [unwired: 2 in, 1 out]
      n65 = Bundle By Name(cluster=w115, "GUID"=w128, "Drop Coords"=w125, "Process Name"=w124) -> (w116:T45)
      n66 = vi-ref "TCU Module.lvlib:TCU Module (Main).vi"() -> (w120:refnum<vi>)
      n67 = property class="VI"(reference=w120) -> ("Path"=w119:path)  [unwired: 1 in, 2 out]
      n68 = Build Array (concatenate)(w122, w116) -> (w121:T45[])
      n69 = To Variant(anything=w116) -> (Variant=w126:variant)
      n70 = Bundle By Name(cluster=w118, "Main Config.TCU Module Configs"=w121) -> (w123:T2)
      n71 = Bundle By Name(cluster=w127, "Module VI Filepath"=w119, "Module Parameters"=w126, "Process Name"=w124) -> (w129:T63)
    }
    frame "TT" {
      (unwired) "TT (Main).vit"  # Filename
      w147 = "TT%d"  # Prefix
      n72 = Unbundle By Name(w132) -> ("Main Config.TT Module Configs"=w139:T33[])
      n73 = Format Into String(format string=w147, w133) -> (resulting string=w141:string)  [unwired: 2 in, 1 out]
      n74 = call "Default Numeric Alarms (TT).vi"() -> ("Default Numeric Alarms"=w131:T65)  [unwired: 11 in]
      n75 = Bundle By Name(cluster=T33 {"GUID"="", "Drop Coords"={"Horizontal"=0, "Vertical"=0}, "Input Channel Tag Name "="", "Process Name"="", "Queue Name"="", "Input Channel Numeric Alarm Settings"=[]} ("TT Module Config"), "GUID"=w145, "Drop Coords"=w142, "Process Name"=w141, "Input Channel Numeric Alarm Settings"=w131) -> (w137:T33)
      n76 = vi-ref "TT (Main).vi"() -> (w135:refnum<vi>)
      n77 = property class="VI"(reference=w135) -> ("Path"=w134:path)  [unwired: 1 in, 2 out]
      n78 = Build Array (concatenate)(w139, w137) -> (w138:T33[])
      n79 = To Variant(anything=w137) -> (Variant=w143:variant)
      n80 = Bundle By Name(cluster=w144, "Module VI Filepath"=w134, "Module Parameters"=w143, "Process Name"=w141) -> (w146:T63)
      n81 = Bundle By Name(cluster=w132, "Main Config.TT Module Configs"=w138) -> (w136:T2)
    }
    frame "U3" {
      (unwired) "U3 (Main).vit"  # Filename
      w164 = "U3%d"  # Prefix
      n82 = Unbundle By Name(w149) -> ("Main Config.U3 Module Configs"=w156:T41[])
      n83 = Format Into String(format string=w164, w150) -> (resulting string=w158:string)  [unwired: 2 in, 1 out]
      n84 = call "Default Numeric Alarms (TT).vi"() -> ("Default Numeric Alarms"=w148:T65)  [unwired: 11 in]
      n85 = Bundle By Name(cluster=T41 {"GUID"="", "Drop Coords"={"Horizontal"=0, "Vertical"=0}, "AI Channel Number"=enum."Default", "Process Name"="", "Queue Name"="", "Input Channel Numeric Alarm Settings"=[]} ("TT Module Config"), "GUID"=w162, "Drop Coords"=w159, "Process Name"=w158, "Input Channel Numeric Alarm Settings"=w148) -> (w154:T41)
      n86 = vi-ref "U3 Module.lvlib:U3 (Main).vit"() -> (w152:refnum<vi>)
      n87 = property class="VI"(reference=w152) -> ("Path"=w151:path)  [unwired: 1 in, 2 out]
      n88 = Build Array (concatenate)(w156, w154) -> (w155:T41[])
      n89 = To Variant(anything=w154) -> (Variant=w160:variant)
      n90 = Bundle By Name(cluster=w161, "Module VI Filepath"=w151, "Module Parameters"=w160, "Process Name"=w158) -> (w163:T63)
      n91 = Bundle By Name(cluster=w149, "Main Config.U3 Module Configs"=w155) -> (w153:T2)
    }
    frame "PT" {
      w181 = "PT%d"  # Process Name
      n92 = Unbundle By Name(w166) -> ("Main Config.PT Module Configs"=w173:T36[])
      n93 = Format Into String(format string=w181, w167) -> (resulting string=w175:string)  [unwired: 2 in, 1 out]
      n94 = call "Default Numeric Alarms (TT).vi"() -> ("Default Numeric Alarms"=w165:T65)  [unwired: 11 in]
      n95 = Bundle By Name(cluster=T36 {"GUID"="", "Drop Coords"={"Horizontal"=0, "Vertical"=0}, "Input Channel Tag Name "="", "Process Name"="", "Queue Name"="", "Input Channel Numeric Alarm Settings"=[]} ("TT Module Config"), "GUID"=w179, "Drop Coords"=w176, "Process Name"=w175, "Input Channel Numeric Alarm Settings"=w165) -> (w171:T36)
      n96 = vi-ref "PT (Main).vi"() -> (w169:refnum<vi>)
      n97 = property class="VI"(reference=w169) -> ("Path"=w168:path)  [unwired: 1 in, 2 out]
      n98 = To Variant(anything=w171) -> (Variant=w177:variant)
      n99 = Build Array (concatenate)(w173, w171) -> (w172:T36[])
      n100 = Bundle By Name(cluster=w178, "Module VI Filepath"=w168, "Module Parameters"=w177, "Process Name"=w175) -> (w180:T63)
      n101 = Bundle By Name(cluster=w166, "Main Config.PT Module Configs"=w172) -> (w170:T2)
    }
    frame "OPC" {
      w197 = "OP%d"  # Process Name
      n102 = Unbundle By Name(w185) -> ("Main Config.OPC Module Configs"=w191:T9[])
      n103 = Format Into String(format string=w197, w186) -> (resulting string=w192:string)  [unwired: 2 in, 1 out]
      n104 = Bundle By Name(cluster=T9 {"State"=enum."Idle", "GUID"="", "Drop Coords"={"Horizontal"=0, "Vertical"=0}, "Configuration"={"Cycle Period"=500.0, "server endpoint URL"="", "security policy"={"message mode"=enum."None", "security"=enum."Basic256"}, "Trust Any Server"=TRUE}, "First Iteration"=FALSE, "Data"=[], "Process Name"="", "Load Count"=0, "Log Started"=FALSE, "subscription ID out"=0, "OPC UA client refnum out"="", "Event Registration Refnum"=refnum, "Start Time"=timestamp(0 s since 1904-01-01), "Current Time"=timestamp(0 s since 1904-01-01)} ("OPC Module Config"), "GUID"=w196, "Drop Coords"=w193, "Process Name"=w192) -> (w189:T9)
      n105 = vi-ref "OPC Main.vi"() -> (w184:refnum<vi>)
      n106 = property class="VI"(reference=w184) -> ("Path"=w187:path)  [unwired: 1 in, 2 out]
      n107 = To Variant(anything=w189) -> (Variant=w194:variant)
      n108 = Build Array (concatenate)(w191, w189) -> (w190:T9[])
      n109 = Bundle By Name(cluster=w195, "Module VI Filepath"=w187, "Module Parameters"=w194, "Process Name"=w192) -> (w182:T63)
      n110 = Bundle By Name(cluster=w185, "Main Config.OPC Module Configs"=w190) -> (w188:T2)
    }
    frame Default {
      # "This case should not execute."
    }
  }
  "Drop Parameters" <- w16
  "State out" <- w2
